vi "OpenCANBus.vi"(8 "Error In":errorcluster, 11 "USB-CAN COM Port":refnum<visa-resource-name>="ASRL3::INSTR") -> (0 "Error Out":errorcluster, 3 "VISA resource name out":refnum<visa-resource-name>)   [LabVIEW 2019, in "CubeMarsBLDClib.lvlib"]
uses:
  CubeMarsBLDClib.lvlib
  <vilib>/myRIO/Instrument Drivers/Onboard IO/UART/typedef/VISA Configuration.ctl
  <vilib>/Instr/_visa.llb/VISA Set IO Buffer Mask.ctl
  <vilib>/Instr/_visa.llb/VISA Configure Serial Port (Instr).vi
  <vilib>/myRIO/Instrument Drivers/Onboard IO/UART/UART.lvlib
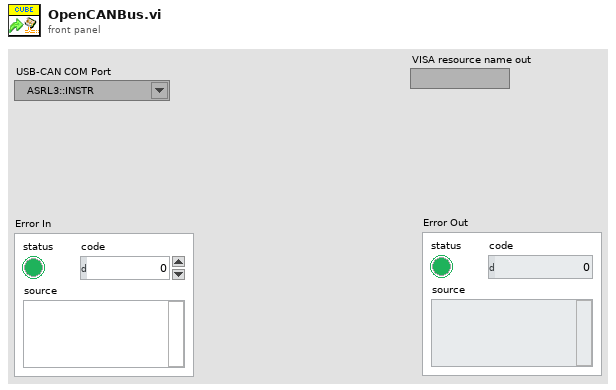
[diagram p1: front panel]
types:
  T1 = typedef "VISA Set IO Buffer Mask.ctl" = u16
  T2 = typedef "UART.lvlib/VISA Configuration.ctl" = cluster{"baud rate (9600)":u32, "data bits (8)":u16, "parity (0:none)":enum16{"None", "Odd", "Even", "Mark", "Space"}, "stop bits (10: 1 bit)":u16, "flow control (0:none)":u16, "termination char\n(0xA = '\\n' = LF) ":u8, "Enable Termination\nChar (T)":bool, "timeout (10sec)":u32}
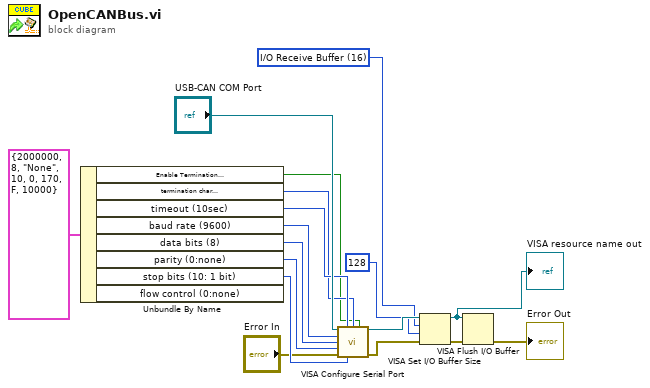
[diagram p0: block diagram]
diagram:
  w4 = T1 16 items=["I/O Receive Buffer"=16, "I/O Transmit Buffer"=32, "I/O Receive and Transmit Buffer"=48] ("Mask")
  n1 = Unbundle By Name(T2 {"baud rate (9600)"=2000000, "data bits (8)"=8, "parity (0:none)"=enum."None", "stop bits (10: 1 bit)"=10, "flow control (0:none)"=0, "termination char\n(0xA = '\\n' = LF) "=170, "Enable Termination\nChar (T)"=FALSE, "timeout (10sec)"=10000} ("VISA Configuration")) -> ("Enable Termination\nChar (T)"=w9:bool, "termination char\n(0xA = '\\n' = LF)"=w10:u8, "timeout (10sec)"=w15:u32, "baud rate (9600)"=w11:u32, "data bits (8)"=w12:u16, "parity (0:none)"=w13:enum16{"None", "Odd", "Even", "Mark", "Space"}, "stop bits (10: 1 bit)"=w14:u16)  [unwired: 1 out]
  n2 = call-poly "VISA Configure Serial Port"("VISA resource name"="USB-CAN COM Port", "timeout (10sec)"=w15, "termination char\n(0xA = '\\n' = LF)"=w10, "Enable Termination\nChar (T)"=w9, "baud rate (9600)"=w11, "data bits (8)"=w12, "parity (0:none)"=w13, "error in (no error)"="Error In", "stop bits (10: 1 bit)"=w14) -> ("VISA resource name out"=w6:refnum<visa-resource-name>, "error out"=w7:errorcluster)  [unwired: 5 in]
  n3 = VISA Set I/O Buffer Size(VISA resource name=w6, mask (16)=w4, size (4096)=u32 128, error in (no error)=w7) -> (VISA resource name out=w3:refnum<visa-resource-name>, error out=w1:errorcluster)
  "VISA resource name out" <- w3
  n4 = VISA Flush I/O Buffer(VISA resource name=w3, error in (no error)=w1) -> (error out=→"Error Out":errorcluster)  [unwired: 1 in, 1 out]
